vi "Shooter_Hood_Untested.vi"() -> ()   [LabVIEW 2019]
uses:
  Control 5.ctl
panel:
  in  "Close_Hood":dbl
  in  "Open_Hood":dbl
  in  "Stop":dbl
  in  "Close_hood":bool
  in  "Open_Hood":bool
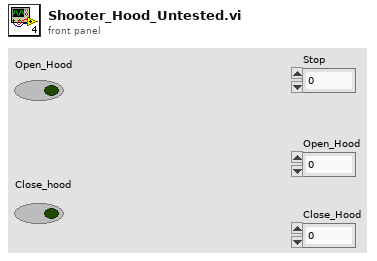
[diagram p1: front panel]
types:
  T1 = typedef "Control 5.ctl" = enum16{"Stop", "Open_Hood", "Close_Hood"}
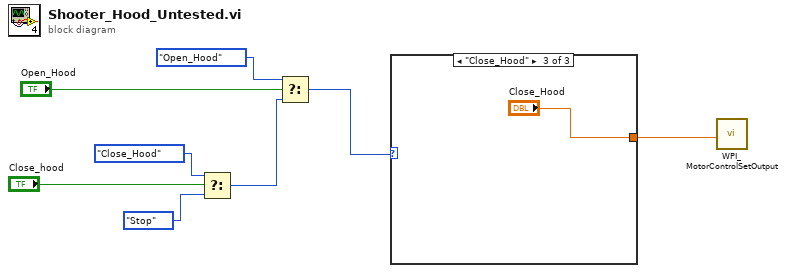
[diagram p0: block diagram]
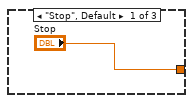
[diagram p2: hidden frame]
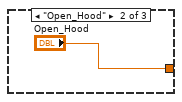
[diagram p3: hidden frame]
diagram:
  n1 = Select(t=Control_5."Close_Hood", s="Close_hood", f=Control_5."Stop") -> (s? t:f=w4:T1)
  n2 = Select(t=Control_5."Open_Hood", s="Open_Hood", f=w4) -> (s? t:f=w2:T1)
  n3 = case shown="\"Close_Hood\"" w2 {
    tunnel: ["Stop" "Open_Hood" "Close_Hood"] -> w1
    frame "Stop", Default {
    }
    frame "Open_Hood" {
    }
    frame "Close_Hood" {
    }
  }
  n4 = call <vilib>:"WPI_MotorControlSetOutput.vi"("Output"=w1) -> ()  [unwired: 8 in, 3 out]
